vi "Find Edge.vi"(8 "error in":errorcluster, 9 "input cluster":T1, 11 "Gantry In":refnum<k24>) -> (0 "error out":errorcluster, 1 "Error?":bool, 3 "Gantry Out":refnum<k24>)   [LabVIEW 2021, in "Component Tray.lvclass"]
uses:
  Workspace/Component/Component Tray.lvclass
  C:/Program Files (x86)/Aerotech/A3200/LabVIEW/2010/Bin/Aerotech.A3200.dll
  Program Files (x86)/Aerotech/A3200/LabVIEW/2010/Bin/Aerotech.A3200.dll
  Workspace/Component/Find Component.ctl
  Camera/Machine Vision.ctl
  A3200.lvclass
  Camera/Camera.lvclass
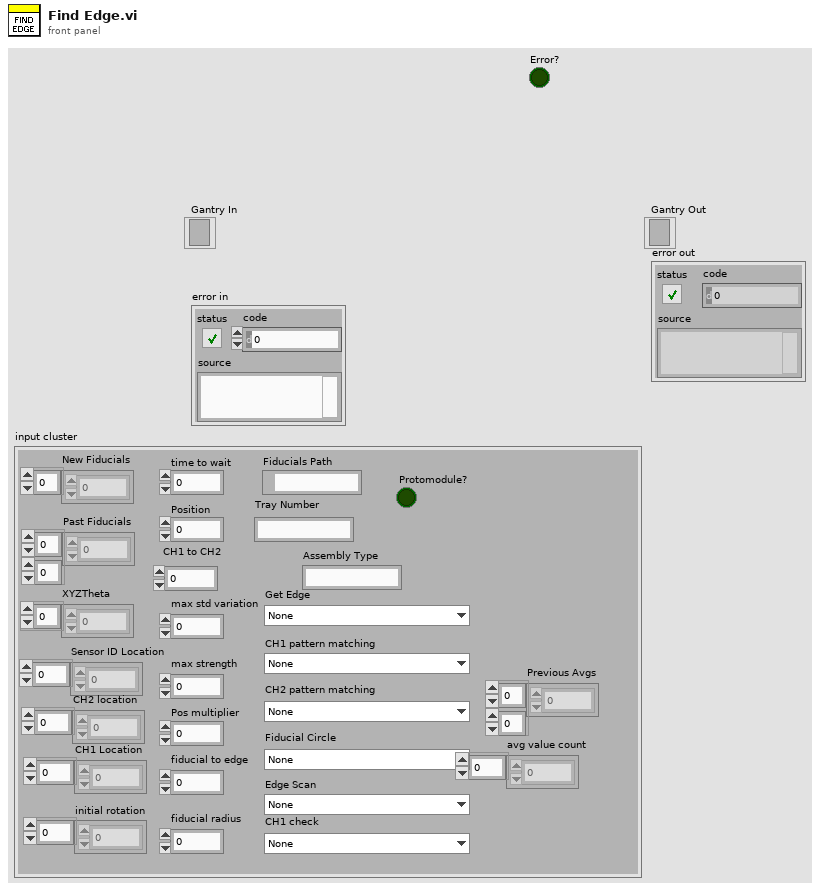
[diagram p1: front panel]
types:
  T1 = typedef "Component Tray.lvclass/Find Component.ctl" = cluster{"New Fiducials":dbl[], "Past Fiducials":dbl[][], "XYZTheta":dbl[], "Fiducials Path":path, "Position":i32, "CH1 Location":dbl[], "Sensor ID Location":dbl[], "initial rotation":dbl[], "CH2 location":dbl[], "max std variation":dbl, "max strength":dbl, "CH2 pattern matching":T2, "Fiducial Circle":T2, "Get Edge":T2, "Pos multiplier":dbl, "time to wait":u32, "fiducial to edge":dbl, "Protomodule?":bool, "Assembly Type":string, "CH1 to CH2":dbl, "Tray Number":string, "fiducial radius":dbl, "4 fiducials?":bool, "CH1 check":T2, "Edge Scan":T2, "CH1 pattern matching":T2, "Sensor Thickness":dbl, "Previous Avgs":dbl[][], "avg value count":dbl[]}
  T2 = typedef "Camera.lvclass/Machine Vision.ctl" = enum16{"None", "Assembly Tray Circle", "Assembly Tray Fiducial", "Partial Hexaboard", "sensor edge init", "HB edge init", "sensor edge pos1", "sensor edge pos2", "HB edge pos1", "HB edge pos2", "Sensor CH1-2", "HB CH1", "HB CH2", "V3 Sensor Circle", "Hexaboard Circle", "sensor CH1 check", "HB CH1 check ", "sensor ID"}
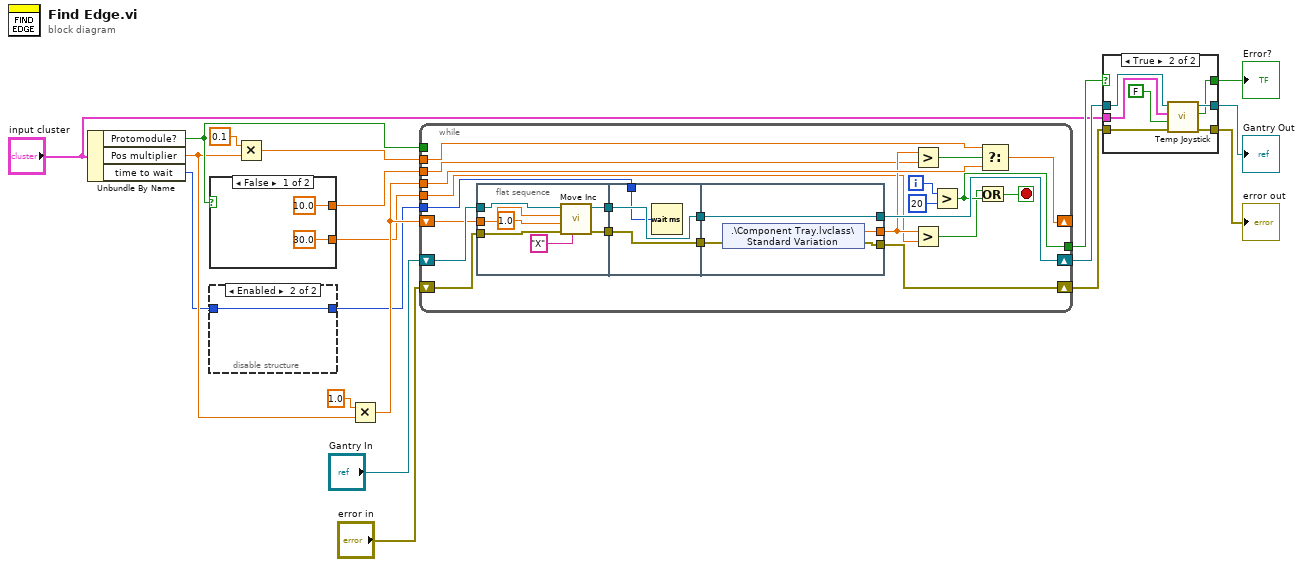
[diagram p0: block diagram]
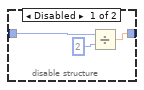
[diagram p2: hidden frame]
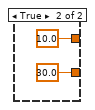
[diagram p4: hidden frame]
diagram:
  n1 = Unbundle By Name("input cluster") -> ("Protomodule?"=w11:bool, "Pos multiplier"=w10:dbl, "time to wait"=w2:u32)
  n2 = case shown="False" w11 {
    tunnel: [sgl 30.0 ("y") sgl 30.0 ("y")] -> w13
    tunnel: [sgl 10.0 ("y") sgl 10.0 ("y")] -> w12
    frame False {
    }
    frame True {
    }
  }
  n3 = disable-structure shown="Enabled" {
    disable-tunnel: w2 -> [w26 w27]
    disable-tunnel: [w24 w27] -> w1
    frame Disabled {
      n4 = Divide(x=w26, y=u32 2) -> (x/y=w24:dbl)
    }
    frame Enabled {
    }
  }
  n5 = Multiply(x=0.1, y=w10) -> (x*y=w14:dbl)
  n6 = Multiply(x=1.0 ("Distance"), y=w10) -> (x*y=w15:dbl)
  n7 = while {
    shift-right: [w46] -> w9
    shift-left: "Gantry In" -> [w49]
    shift-right: [w42] -> w8
    shift-left: "error in" -> [w45]
    shift-right: [w37] -> _
    shift-left: w15 -> [w40]
    tunnel: w15 -> [w38]
    tunnel: w14 -> [w39]
    tunnel: w13 -> [w35]
    tunnel: w12 -> [w34]
    tunnel: w11 -> [_]
    tunnel: [w30] -> w7
    tunnel: w1 -> [w29]
    i -> [w32]
    stop <- w33 stop-if-true
    n8 = flat-sequence {
      tunnel: w49 -> [w54]
      tunnel: [w53] -> w47
      tunnel: w45 -> [w52]
      tunnel: [w51] -> w43
      tunnel: w40 -> [w50]
      tunnel: [w59] -> w48
      tunnel: w47 -> [w59]
      tunnel: [w58] -> w44
      tunnel: w43 -> [w58]
      tunnel: w29 -> [w57]
      tunnel: [w63] -> w46
      tunnel: w48 -> [w63]
      tunnel: w44 -> [w61]
      tunnel: [w60] -> w42
      tunnel: [w62] -> w36
      frame #0 {
        n9 = call "Move Inc.vi"("Axis"="X", "error in (no error)"=w52, "Speed"=1.0, "Distance"=w50, "Gantry In"=w54) -> ("error out"=w51:errorcluster, "Gantry Out"=w53:refnum<k24>)  [unwired: 5 in]
      }
      frame #1 {
        n10 = Wait (ms)(milliseconds to wait=w57) -> ()  [unwired: 1 out]
      }
      frame #2 {
        n11 = shared-variable ".\\Component Tray.lvclass\\Standard Variation"(error in=w61) -> (w62:sgl, error out=w60:errorcluster)
      }
    }
    n12 = Greater?(x=w36, y=w34) -> (0:w41:bool)
    n13 = Greater?(x=w36, y=w35) -> (0:w28:bool)
    n14 = Greater?(x=w32, y=20) -> (0:w30:bool)
    n15 = Or(x=w28, y=w30) -> (x .or. y?=w33:bool)
    n16 = Select(t=w39, s=w41, f=w38) -> (s? t:f=w37:dbl)
  }
  n17 = case shown="True" w7 {
    selector: w7 -> [w64 _]
    tunnel: w9 -> [w66 w73]
    tunnel: [w66 w72] -> w6
    tunnel: "input cluster" -> [_ w71]
    tunnel: w8 -> [w65 w69]
    tunnel: [w65 w68] -> w4
    tunnel: [w64 w67] -> w3
    frame False {
    }
    frame True {
      n18 = call "Temp Joystick.vi"("error in (no error)"=w69, "Fiducial?"=FALSE, "Component"=w71, "Gantry In"=w73) -> ("error out"=w68:errorcluster, "Error?"=w67:bool, "Gantry Out"=w72:refnum<k24>)  [unwired: 5 in]
    }
  }
  "Gantry Out" <- w6
  "error out" <- w4
  "Error?" <- w3
